vi "Handle Error.vi"(8 "error in (no error)":errorcluster, 11 "Base UI Actor in":refnum<class "Base UI Actor.lvclass">) -> (0 "error out":errorcluster, 2 "stop actor?":bool=TRUE, 3 "Base UI Actor out":refnum<class "Base UI Actor.lvclass">)   [LabVIEW 2016, in "Assert API Components.lvlib" / "Base UI Actor.lvlib" / "Base UI Actor.lvclass"]
doc: "(<B>Filename</B>: Actor Framework.lvlib:Actor.lvclass:Handle Error.vi)\n\nDefines how the actor handles an error that occurred while processing a message. By default, this method does nothing except stop the actor."
uses:
  Base UI Actor.lvclass
  <vilib>/Utility/sysdir.llb/System Directory Type.ctl
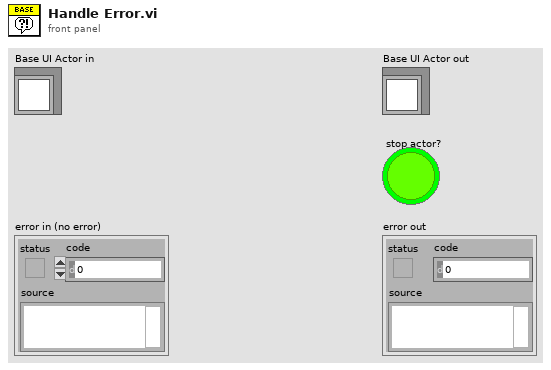
[diagram p1: front panel]
types:
  T1 = enum16{"open", "replace", "create", "open or create", "replace or create", "replace or create with confirmation"}
  T2 = typedef "System Directory Type.ctl" = i32
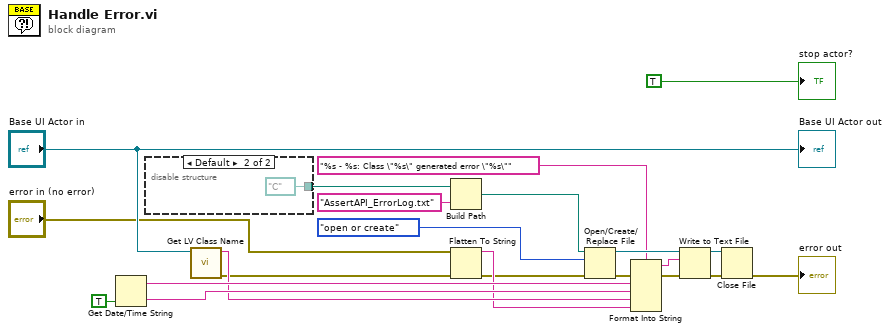
[diagram p0: block diagram]
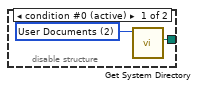
[diagram p2: hidden frame]
diagram:
  n1 = Get Date/Time String(want seconds? (F)=TRUE) -> (date string=w19:string, time string=w18:string)  [unwired: 2 in]
  n2 = disable-structure shown="Default" {
    disable-tunnel: [w23 path "C:/" ("system directory")] -> w9
    frame condition #0 (active) {
      w24 = T2 2 items=["User Home"=0, "User Desktop"=1, "User Documents"=2, "User Application Data"=3, "User Preferences"=4, "User Temporary"=5, "Public Documents"=6, "Public Application Data"=7, "Public Preferences"=8, "Public Cache"=13, "System Core Libraries"=9, "System Installed Libraries"=10, "Application Files"=11, "Boot Volume Root"=12] ("system directory type")
      n3 = call <vilib>:"Get System Directory.vi"("system directory type"=w24) -> ("system directory"=w23:path)  [unwired: 10 in]
    }
    frame condition #1 {
    }
  }
  n4 = call <vilib>:"Get LV Class Name.vi"("object"="Base UI Actor in") -> ("error out"=w15:errorcluster, "class name"=w16:string)  [unwired: 9 in]
  n5 = Build Path(base path=w9, name or relative path="AssertAPI_ErrorLog.txt") -> (appended path=w7:path)
  n6 = Flatten To String(anything="error in (no error)", error in (no error)=w15) -> (data string=w10:string, error out=w5:errorcluster)  [unwired: 2 in, 1 out]
  n7 = Open/Create/Replace File(file path (use dialog)=w7, error in=w5, operation (0:open)=T1."open or create") -> (refnum out=w12:refnum<file>, error out=w4:errorcluster)  [unwired: 3 in, 1 out]
  n8 = Format Into String(format string="%s - %s: Class \"%s\" generated error \"%s\"", error in=w4, w19, w18, w16, w10) -> (resulting string=w6:string, error out=w3:errorcluster)  [unwired: 1 in]
  n9 = Write to Text File(file (use dialog)=w12, text=w6, error in=w3) -> (refnum out=w11:refnum<file>, error out=w14:errorcluster)  [unwired: 1 in, 1 out]
  n10 = Close File(refnum=w11, error in=w14) -> (error out=→"error out":errorcluster)  [unwired: 1 out]
  "Base UI Actor out" <- "Base UI Actor in"
  "stop actor?" <- TRUE ("stop actor?")
